vi "Get-latest-map.vi"(8 "error in (no error)":errorcluster, 10 "UI ref. in":refnum<data-value>, 11 "Data ref. in":refnum<data-value>) -> (0 "error out":errorcluster, 1 "2D map":dbl[][](array[numeric]), 2 "UI ref.":refnum<data-value>, 3 "Data ref.":refnum<data-value>)   [LabVIEW 2013, in "CameraVision.lvlib" / "CV-Main.lvclass"]
uses:
  CV-Main.lvclass
  UI/CV-UI.lvclass
  UI/CV-UI.lvclass/CV-UI.ctl
  CV-Main.lvclass/CV-Main.ctl
  UI/Read Camera.vi
  UI/Read Mapping-characteristic.vi
  Read Map.vi
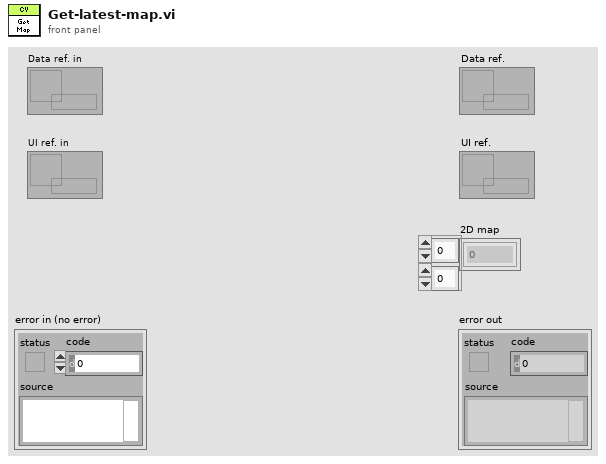
[diagram p1: front panel]
types:
  T1 = typedef "CameraVision.lvlib/CV-Mapping.lvclass/Mapping-characteristic.ctl" = enum16{"Average intensity [0-255]", "Peak intensity [0-255]", "Melt-pool size [mm²]", "Melt-pool aspect ratio []", "Melt-pool fragments []", "Average temperature [°C]", "Max. temperature [°C]", "Min. temperature [°C]", "Std. dev. temperature [°C]"}
  T2 = typedef "CameraVision.lvlib/CV-Buffers.lvclass/Mapping-buffer.ctl" = cluster{"Time":timestamp, "Index":i32, "Temperature characteristics":T3, "Characteristics":T4[], "Xcoord":sgl, "Ycoord":sgl}
  T3 = typedef "CameraVision.lvlib/CV-Temperature.lvclass/Temperature-characteristics.ctl" = cluster{"Average temperature ":dbl, "Max. temperature":dbl, "Min. temperature":dbl, "Stand. dev. temperature":dbl, "Datapoints":dbl}
  T4 = typedef "CameraVision.lvlib/CV-Analysis.lvclass/Characteristics-cluster.ctl" = cluster{"Average intensity":dbl, "Peak intensity":dbl, "Melt-pool size":dbl, "Melt-pool aspect ratio":dbl, "Melt-pool fragments":dbl, "Centre of mass X":dbl, "Centre of mass Y":dbl, "Orientation":dbl}
  T5 = typedef "CameraVision.lvlib/CV-UI.lvclass/Camera-selector.ctl" = enum16{"Camera 1", "Camera 2"}
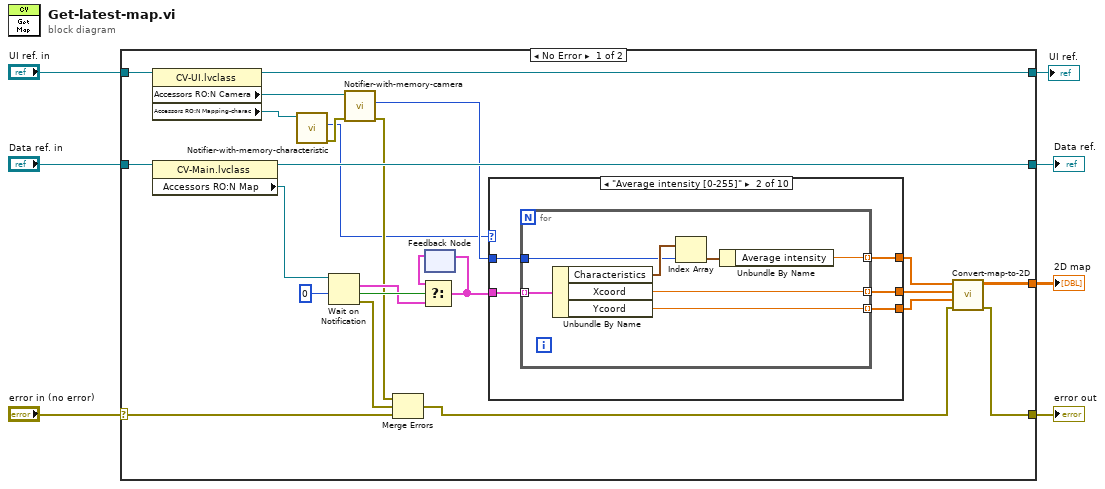
[diagram p0: block diagram]
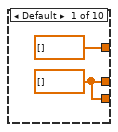
[diagram p2: hidden frame]
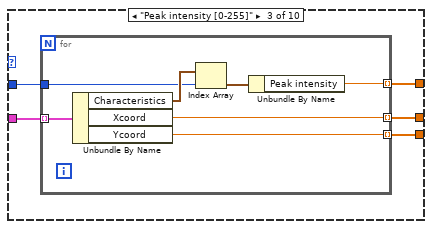
[diagram p3: hidden frame]
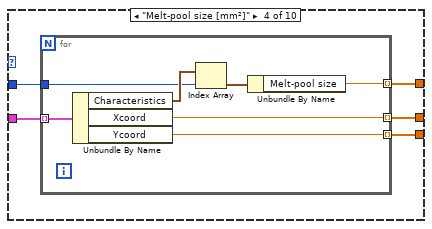
[diagram p4: hidden frame]
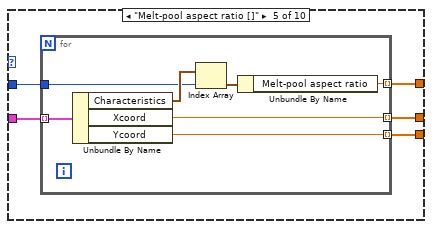
[diagram p5: hidden frame]
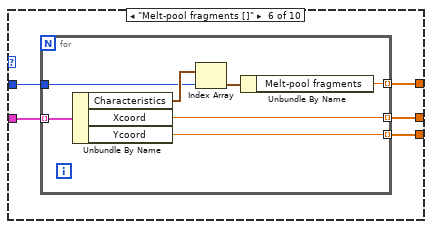
[diagram p6: hidden frame]
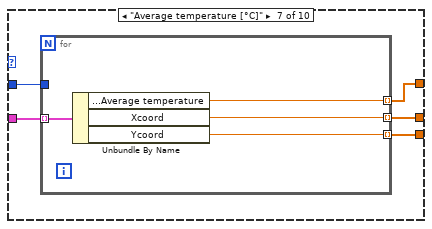
[diagram p7: hidden frame]
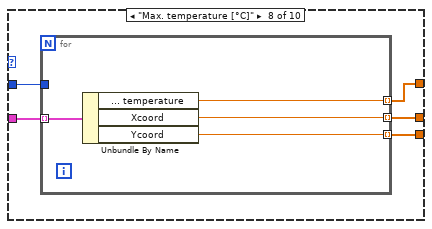
[diagram p8: hidden frame]
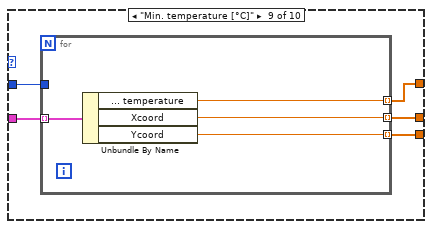
[diagram p9: hidden frame]
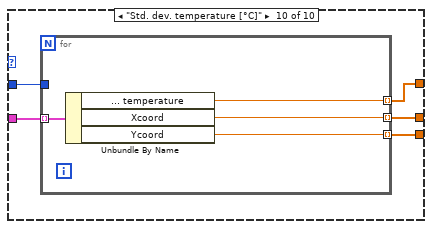
[diagram p10: hidden frame]
diagram:
  n1 = case shown="No Error" "error in (no error)" {
    selector: "error in (no error)" -> [w23 w132]
    tunnel: [w10 w132] -> w6
    tunnel: "Data ref. in" -> [w31 w131]
    tunnel: [w30 w131] -> w4
    tunnel: "UI ref. in" -> [w22 w130]
    tunnel: [w9 w130] -> w2
    tunnel: [w8 _] -> w1
    frame No Error {
      n2 = property class="CV-UI.lvclass"(reference=w22) -> (reference out=w9:refnum<data-value>, "Accessors RO:N Camera"=w19:refnum<notifier>, "Accessors RO:N Mapping-charac"=w20:refnum<notifier>)  [unwired: 1 in, 1 out]
      n3 = property class="CV-Main.lvclass"(reference=w31) -> (reference out=w30:refnum<data-value>, "Accessors RO:N Map"=w29:refnum<notifier>)  [unwired: 1 in, 1 out]
      n4 = call "Notifier-with-memory-characteristic.vi"("Notifier in"=w20) -> ("error IO"=w18:errorcluster, "Notification"=w15:T1)  [unwired: 9 in]
      n5 = Wait on Notification(notifier=w29, timeout in ms (-1)=0) -> (notification=w25:T2[], timed out?=w26:bool, error out=w24:errorcluster)  [unwired: 2 in, 1 out]
      n6 = call "Notifier-with-memory-camera.vi"("error in"=w18, "Notifier in"=w19) -> ("error IO"=w17:errorcluster, "Notification"=w16:T5)  [unwired: 8 in]
      n7 = Merge Errors(w17, w24, w23) -> (w11:errorcluster)
      n8 = feedback #1() -> (w27:T2[])  [unwired: 1 in]
      n9 = Select(t=w27, s=w26, f=w25) -> (s? t:f=w21:T2[])
      n10 = feedback-in #1(w21) -> ()
      n11 = case shown="\"Average intensity [0-255]\"" w15 {
        tunnel: w21 -> [_ w38 w50 w62 w74 w86 w98 w107 w116 w125]
        tunnel: w16 -> [_ w37 w49 w61 w73 w85 w97 w106 w115 w124]
        tunnel: [dbl[] [] w36 w48 w60 w72 w84 w96 w105 w114 w123] -> w14
        tunnel: [w33 w35 w47 w59 w71 w83 w95 w104 w113 w122] -> w13
        tunnel: [w33 w34 w46 w58 w70 w82 w94 w103 w112 w121] -> w12
        frame Default {
          w33 = sgl[] []
        }
        frame "Average intensity [0-255]" {
          n12 = for {
            tunnel: w38 -> [w45] mode=indexing
            tunnel: w37 -> [w43]
            tunnel: [w41] -> w36 mode=indexing
            tunnel: [w40] -> w35 mode=indexing
            tunnel: [w39] -> w34 mode=indexing
            n13 = Unbundle By Name(w45) -> ("Characteristics"=w44:T4[], "Xcoord"=w40:sgl, "Ycoord"=w39:sgl)
            n14 = Index Array(array=w44, index=w43) -> (element=w42:T4)
            n15 = Unbundle By Name(w42) -> ("Average intensity"=w41:dbl)
          }
        }
        frame "Peak intensity [0-255]" {
          n16 = for {
            tunnel: w50 -> [w57] mode=indexing
            tunnel: w49 -> [w55]
            tunnel: [w53] -> w48 mode=indexing
            tunnel: [w52] -> w47 mode=indexing
            tunnel: [w51] -> w46 mode=indexing
            n17 = Unbundle By Name(w57) -> ("Characteristics"=w56:T4[], "Xcoord"=w52:sgl, "Ycoord"=w51:sgl)
            n18 = Index Array(array=w56, index=w55) -> (element=w54:T4)
            n19 = Unbundle By Name(w54) -> ("Peak intensity"=w53:dbl)
          }
        }
        frame "Melt-pool size [mm²]" {
          n20 = for {
            tunnel: w62 -> [w69] mode=indexing
            tunnel: w61 -> [w67]
            tunnel: [w65] -> w60 mode=indexing
            tunnel: [w64] -> w59 mode=indexing
            tunnel: [w63] -> w58 mode=indexing
            n21 = Unbundle By Name(w69) -> ("Characteristics"=w68:T4[], "Xcoord"=w64:sgl, "Ycoord"=w63:sgl)
            n22 = Index Array(array=w68, index=w67) -> (element=w66:T4)
            n23 = Unbundle By Name(w66) -> ("Melt-pool size"=w65:dbl)
          }
        }
        frame "Melt-pool aspect ratio []" {
          n24 = for {
            tunnel: w74 -> [w81] mode=indexing
            tunnel: w73 -> [w79]
            tunnel: [w77] -> w72 mode=indexing
            tunnel: [w76] -> w71 mode=indexing
            tunnel: [w75] -> w70 mode=indexing
            n25 = Unbundle By Name(w81) -> ("Characteristics"=w80:T4[], "Xcoord"=w76:sgl, "Ycoord"=w75:sgl)
            n26 = Index Array(array=w80, index=w79) -> (element=w78:T4)
            n27 = Unbundle By Name(w78) -> ("Melt-pool aspect ratio"=w77:dbl)
          }
        }
        frame "Melt-pool fragments []" {
          n28 = for {
            tunnel: w86 -> [w93] mode=indexing
            tunnel: w85 -> [w91]
            tunnel: [w89] -> w84 mode=indexing
            tunnel: [w88] -> w83 mode=indexing
            tunnel: [w87] -> w82 mode=indexing
            n29 = Unbundle By Name(w93) -> ("Characteristics"=w92:T4[], "Xcoord"=w88:sgl, "Ycoord"=w87:sgl)
            n30 = Index Array(array=w92, index=w91) -> (element=w90:T4)
            n31 = Unbundle By Name(w90) -> ("Melt-pool fragments"=w89:dbl)
          }
        }
        frame "Average temperature [°C]" {
          n32 = for {
            tunnel: w98 -> [w102] mode=indexing
            tunnel: w97 -> [_]
            tunnel: [w99] -> w96 mode=indexing
            tunnel: [w101] -> w95 mode=indexing
            tunnel: [w100] -> w94 mode=indexing
            n33 = Unbundle By Name(w102) -> ("Temperature characteristics.Average temperature"=w99:dbl, "Xcoord"=w101:sgl, "Ycoord"=w100:sgl)
          }
        }
        frame "Max. temperature [°C]" {
          n34 = for {
            tunnel: w107 -> [w111] mode=indexing
            tunnel: w106 -> [_]
            tunnel: [w108] -> w105 mode=indexing
            tunnel: [w110] -> w104 mode=indexing
            tunnel: [w109] -> w103 mode=indexing
            n35 = Unbundle By Name(w111) -> ("Temperature characteristics.Max. temperature"=w108:dbl, "Xcoord"=w110:sgl, "Ycoord"=w109:sgl)
          }
        }
        frame "Min. temperature [°C]" {
          n36 = for {
            tunnel: w116 -> [w120] mode=indexing
            tunnel: w115 -> [_]
            tunnel: [w117] -> w114 mode=indexing
            tunnel: [w119] -> w113 mode=indexing
            tunnel: [w118] -> w112 mode=indexing
            n37 = Unbundle By Name(w120) -> ("Temperature characteristics.Min. temperature"=w117:dbl, "Xcoord"=w119:sgl, "Ycoord"=w118:sgl)
          }
        }
        frame "Std. dev. temperature [°C]" {
          n38 = for {
            tunnel: w125 -> [w129] mode=indexing
            tunnel: w124 -> [_]
            tunnel: [w126] -> w123 mode=indexing
            tunnel: [w128] -> w122 mode=indexing
            tunnel: [w127] -> w121 mode=indexing
            n39 = Unbundle By Name(w129) -> ("Temperature characteristics.Stand. dev. temperature"=w126:dbl, "Xcoord"=w128:sgl, "Ycoord"=w127:sgl)
          }
        }
      }
      n40 = call "Convert-map-to-2D.vi"("error in"=w11, "Ycoords"=w12, "Xcoords"=w13, "Signal"=w14) -> ("error IO"=w10:errorcluster, "2D map"=w8:dbl[][])  [unwired: 6 in]
    }
    frame Error {
    }
  }
  "error out" <- w6
  "Data ref." <- w4
  "UI ref." <- w2
  "2D map" <- w1
